vi "getAdditionalDataFromXMLNative.vi"(8 "error in (no error)":errorcluster, 10 "eventXML":refnum<k20>, 11 "RampEvent in":refnum<class "RampEvent.lvclass">) -> (0 "error out":errorcluster, 2 "eventXML out":refnum<k20>, 3 "RampEvent out":refnum<class "RampEvent.lvclass">)   [LabVIEW 2009, in "Tools.lvlib" / "Scripting.lvlib" / "RampEvent.lvclass"]
uses:
  RampEvent.lvclass
  <vilib>/xml/Close Reference(Node).vi
  RampEvent.lvclass/RampEvent.ctl
  <vilib>/xml/NI_XML.lvlib
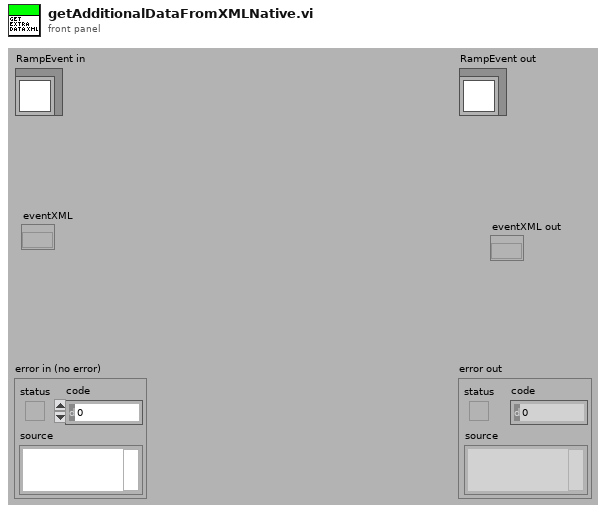
[diagram p1: front panel]
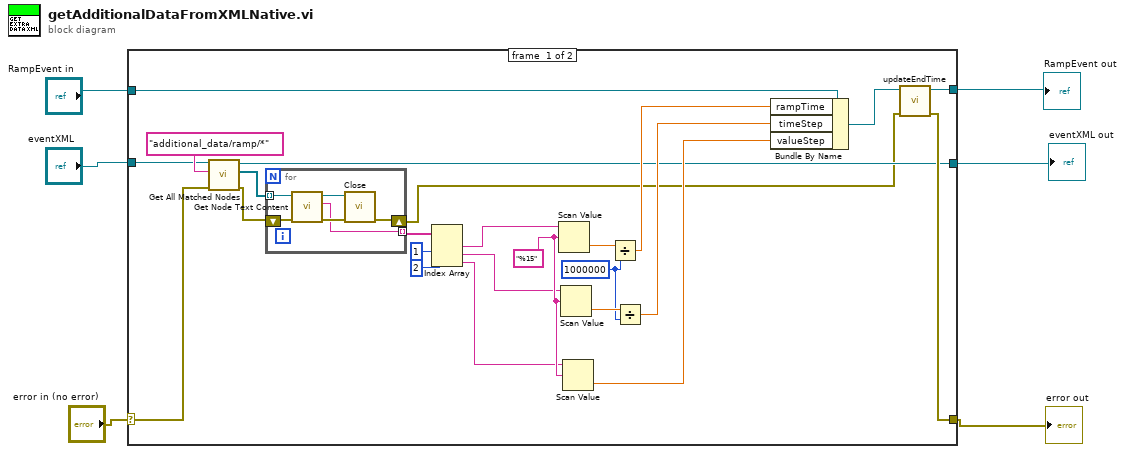
[diagram p0: block diagram]
diagram:
  n1 = case shown="No Error" "error in (no error)" {
    selector: "error in (no error)" -> [w13 w37]
    tunnel: [w20 w37] -> w3
    tunnel: "RampEvent in" -> [w25 w38]
    tunnel: [w21 w38] -> w4
    tunnel: "eventXML" -> [w14 _]
    tunnel: [w12 _] -> w1
    frame #0 {
      w28 = 1000000
      w24 = "%15"
      n2 = call <vilib>:"Get All Matched Nodes.vi"("error in (no error)"=w13, "XPath expression"="additional_data/ramp/*", "node in"=w14) -> ("error out"=w19:errorcluster, "node result array"=w17:refnum<k20>[], "node out"=w12:refnum<k20>)  [unwired: 6 in]
      n3 = for {
        tunnel: w17 -> [w33] mode=indexing
        tunnel: [w32] -> w16 mode=indexing
        shift-right: [w31] -> w7
        shift-left: w19 -> [w34]
        n4 = call <vilib>:"Get Node Text Content.vi"("error in (no error)"=w34, "node in"=w33) -> ("error out"=w35:errorcluster, "node text"=w32:string, "node out"=w36:refnum<k20>)  [unwired: 7 in]
        n5 = call-poly <vilib>:"Close.vi"("error in (no error)"=w35, "node"=w36) -> ("error out"=w31:errorcluster)  [unwired: 7 in]
      }
      n6 = Index Array(array=w16, index #2=1 ("index"), index #3=2 ("index")) -> (element #1=w10:string, element #2=w9:string, element #3=w8:string)  [unwired: 1 in]
      n7 = Scan Value(string=w10, format string=w24) -> (value=w30:dbl)  [unwired: 1 in, 1 out]
      n8 = Scan Value(string=w9, format string=w24) -> (value=w29:dbl)  [unwired: 1 in, 1 out]
      n9 = Scan Value(string=w8, format string=w24) -> (value=w23:dbl)  [unwired: 1 in, 1 out]
      n10 = Divide(x=w30, y=w28) -> (x/y=w27:dbl)
      n11 = Divide(x=w29, y=w28) -> (x/y=w26:dbl)
      n12 = Bundle By Name(cluster=w25, "rampTime"=w27, "timeStep"=w26, "valueStep"=w23) -> (w22:refnum<class "RampEvent.lvclass">)
      n13 = call-dynamic "updateEndTime.vi"("error in (no error)"=w7, "RampEvent in"=w22) -> ("error out"=w20:errorcluster, "RampEvent out"=w21:refnum<class "RampEvent.lvclass">)  [unwired: 8 in]
    }
    frame #1 {
    }
  }
  "error out" <- w3
  "RampEvent out" <- w4
  "eventXML out" <- w1
